vi "RemoveJump.vi"(9 "frame size":i32, 10 "Input":csg[](array[numeric])) -> (2 "Output":csg[](array[numeric]))   [LabVIEW 2022 SP3]
panel:
  out "Waveform Graph 2":sgl[][](graph)
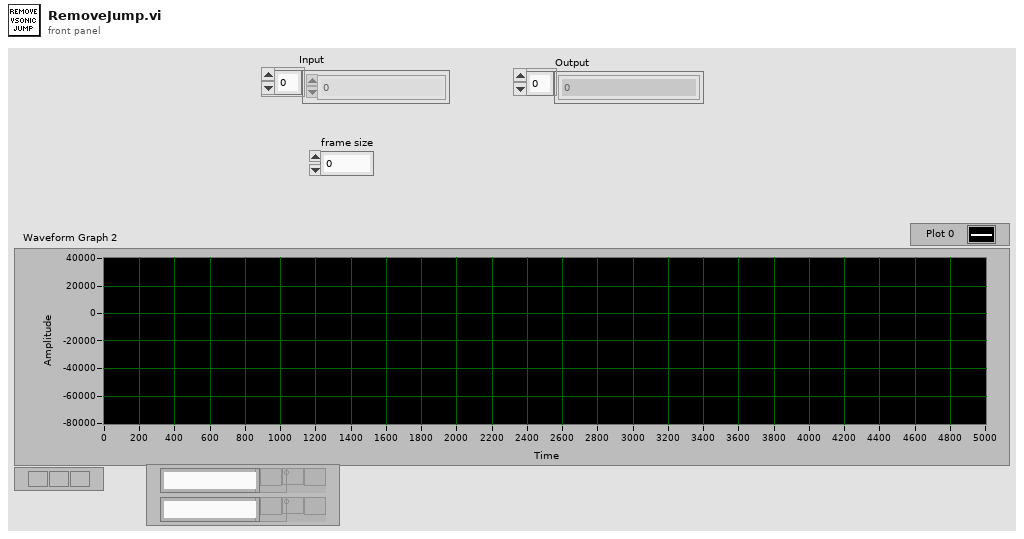
[diagram p1: front panel]
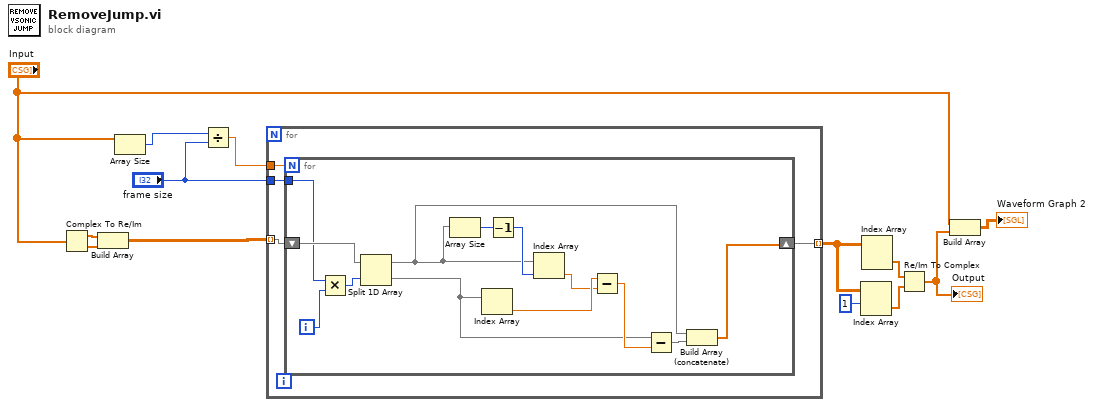
[diagram p0: block diagram]
diagram:
  n1 = Complex To Re/Im(x + iy="Input") -> (x=w12:sgl[], y=w11:sgl[])
  n2 = Build Array(w12, w11) -> (w10:sgl[][])
  n3 = Array Size(array="Input") -> (size(s)=w3:i32)
  n4 = Divide(x=w3, y="frame size") -> (x/y=w1:dbl)
  n5 = for {
    tunnel: [w14] -> w9 mode=indexing
    tunnel: w10 -> [w17] mode=indexing
    tunnel: "frame size" -> [w16]
    tunnel: w1 -> [w15]
    n6 = for {
      N: w15 -> [_]
      shift-right: [w21] -> w14
      shift-left: w17 -> [w22]
      tunnel: w16 -> [w18]
      i -> [w19]
      n7 = Multiply(x=w18, y=w19) -> (x*y=w20:i32)
      n8 = Split 1D Array(array=w22, index=w20) -> (first subarray=w23:sgl[], second subarray=w25:sgl[])
      n9 = Array Size(array=w23) -> (size(s)=w30:i32)
      n10 = Index Array(array=w25) -> (element=w28:sgl)  [unwired: 1 in]
      n11 = Decrement(x=w30) -> (x-1=w29:i32)
      n12 = Index Array(array=w23, index=w29) -> (element=w27:sgl)
      n13 = Subtract(x=w28, y=w27) -> (x-y=w26:sgl)
      n14 = Subtract(x=w25, y=w26) -> (x-y=w24:sgl[])
      n15 = Build Array (concatenate)(w23, w24) -> (w21:sgl[])
    }
  }
  n16 = Index Array(array=w9, index (row)=1) -> (element=w6:sgl[])  [unwired: 1 in]
  n17 = Index Array(array=w9) -> (element=w7:sgl[])  [unwired: 2 in]
  n18 = Re/Im To Complex(1:w6, 2:w7) -> (0:w5:csg[])
  "Output" <- w5
  n19 = Build Array("Input", w5) -> (→"Waveform Graph 2":csg[][])
